vi "Ini_SetOutput.vi"(8 "error in (no error)":errorcluster, 11 "16InOut in":refnum<class "16InOut.lvclass">) -> (0 "error out":errorcluster, 3 "16InOut out":refnum<class "16InOut.lvclass">)   [LabVIEW 2019, in "16InOut.lvclass"]
uses:
  16InOut.lvclass
  IOCard.lvclass/IOCard.ctl
  IOCard.lvclass
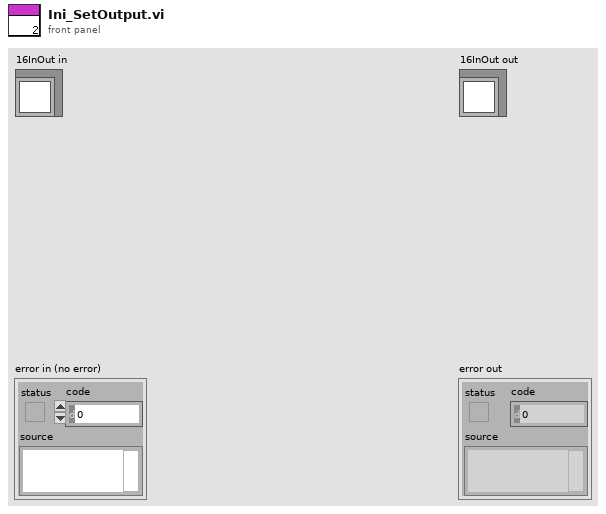
[diagram p1: front panel]
types:
  T1 = typedef "IO Card_Type.ctl" = enum16{"None", "Unidaq32", "6480", "2410C-64", "Zan", "DMC1000B", "16InOut", "Robot", "DMC3600"}
  T2 = cluster{"IO Card Type":T1, "IOType":enum16{"Input", "Output"}, "CardNumber":i32, "ConnectAct":bool, "IP":string}
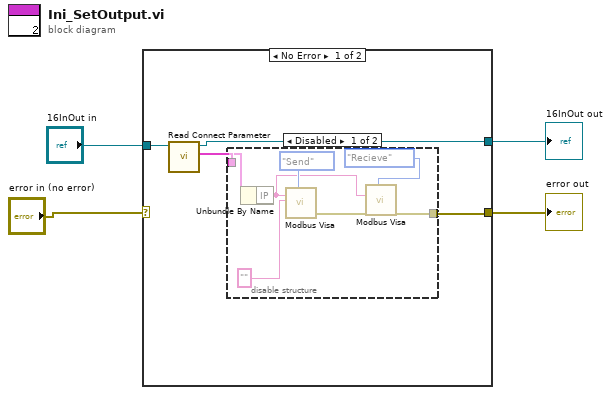
[diagram p0: block diagram]
diagram:
  n1 = case shown="No Error" "error in (no error)" {
    selector: "error in (no error)" -> [_ w16]
    tunnel: "16InOut in" -> [w8 w17]
    tunnel: [w6 w17] -> w2
    tunnel: [w5 w16] -> w1
    frame No Error {
      n2 = call "Read Connect Parameter.vi"("IOCard in"=w8) -> ("Connect Parameter"=w7:T2, "IOCard out"=w6:refnum<class "16InOut.lvclass">)  [unwired: 8 in, 1 out]
      n3 = disable-structure shown="Disabled" {
        disable-tunnel: w7 -> [w15 _]
        disable-tunnel: [w9 _] -> w5
        frame Disabled {
          n4 = Unbundle By Name(w15) -> ("IP"=w12:string)
          n5 = call "Modbus Visa.vi"("VISA resource name"=w12, "Cmd"="", "VisaAction"=enum16{"Open", "Send", "Recieve", "Close"}."Send") -> ("error out"=w11:errorcluster)  [unwired: 15 in, 1 out]
          n6 = call "Modbus Visa.vi"("VISA resource name"=w12, "error in (no error)"=w11, "VisaAction"=enum16{"Open", "Send", "Recieve", "Close"}."Recieve") -> ("error out"=w9:errorcluster)  [unwired: 15 in, 1 out]
        }
        frame Enabled {
        }
      }
    }
    frame Error {
    }
  }
  "error out" <- w1
  "16InOut out" <- w2
